vi "Store Nested Object Queue.vi"(8 "error in (no error)":errorcluster, 9 "Caller-To-Actor Enqueuer":refnum<class "Message Enqueuer.lvclass">, 10 "name":string, 11 "Mag Lab Measure Base in":refnum<class "Mag Lab Measure Base.lvclass">) -> (0 "error out":errorcluster, 3 "Mag Lab Measure Base out":refnum<class "Mag Lab Measure Base.lvclass">)   [LabVIEW 2015, in "Mag Lab Measure Base.lvclass"]
uses:
  Mag Lab Measure Base.lvclass
  <vilib>/ActorFramework/Message Enqueuer/Message Enqueuer.lvclass
  Mag Lab Measure Base.lvclass/Mag Lab Measure Base.ctl
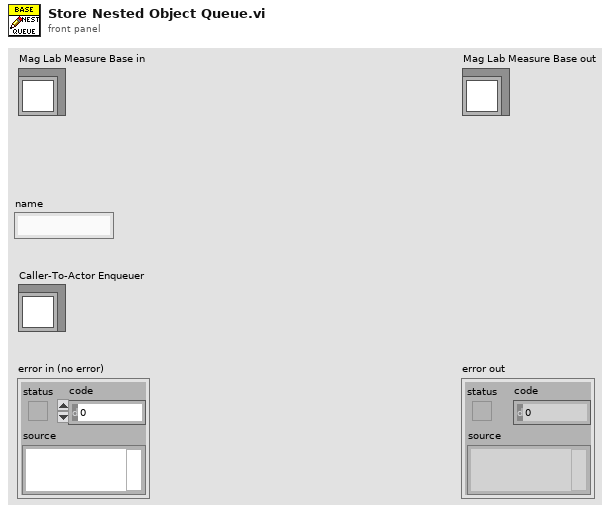
[diagram p1: front panel]
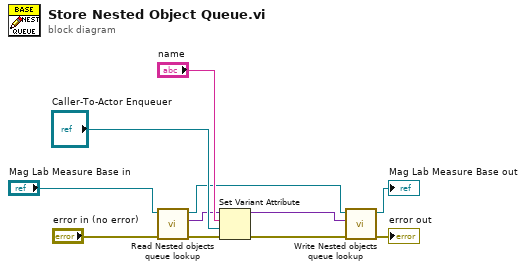
[diagram p0: block diagram]
diagram:
  n1 = call "Read Nested objects queue lookup.vi"("error in (no error)"="error in (no error)", "Mag Lab Measure Base in"="Mag Lab Measure Base in") -> ("error out"=w3:errorcluster, "Nested objects queue lookup"=w8:variant, "Mag Lab Measure Base out"=w7:refnum<class "Mag Lab Measure Base.lvclass">)  [unwired: 7 in]
  n2 = Set Variant Attribute(Variant=w8, name="name", value="Caller-To-Actor Enqueuer", error in=w3) -> (Variant out=w5:variant, error out=w2:errorcluster)  [unwired: 1 out]
  n3 = call "Write Nested objects queue lookup.vi"("error in (no error)"=w2, "Nested objects queue lookup"=w5, "Mag Lab Measure Base in"=w7) -> ("error out"=→"error out":errorcluster, "Mag Lab Measure Base out"=→"Mag Lab Measure Base out":refnum<class "Mag Lab Measure Base.lvclass">)  [unwired: 7 in]
